vi "BuildPieceArrayFromPosition.vi"(8 "error in (no error)":errorcluster, 11 "object in":refnum<class "Board.lvclass">) -> (0 "error out":errorcluster, 3 "object out":refnum<class "Board.lvclass">)   [LabVIEW 2020, in "Board.lvclass"]
doc: "Returns a piece array from the board string"
uses:
  Board.lvclass
  Pieces/typedefs/pieceType.ctl
  Pieces/Piece.lvclass
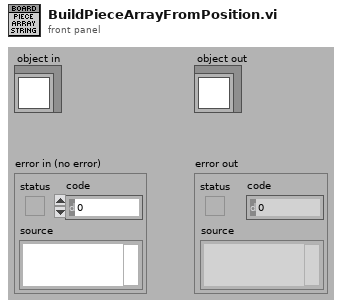
[diagram p1: front panel]
types:
  T1 = typedef "Piece.lvclass/pieceType.ctl" = enum16{"K", "Q", "R", "N", "B", "P", "none"}
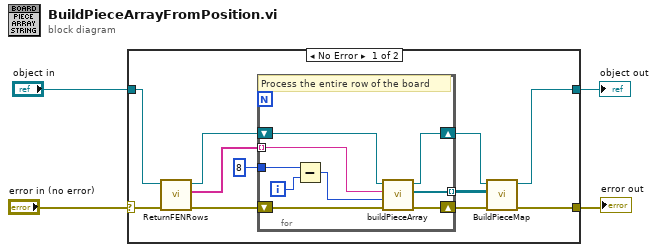
[diagram p0: block diagram]
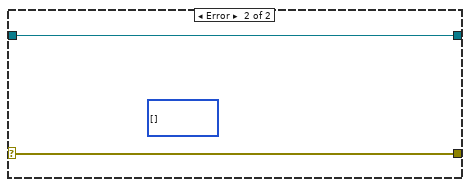
[diagram p2: hidden frame]
diagram:
  n1 = case shown="No Error" "error in (no error)" {
    selector: "error in (no error)" -> [w12 w26]
    tunnel: [w8 w26] -> w3
    tunnel: [w7 w25] -> w1
    tunnel: "object in" -> [w11 w25]
    frame No Error {
      n2 = call "ReturnFENRows.vi"("error in (no error)"=w12, "Board in"=w11) -> ("error out"=w13:errorcluster, "StandardPieceLocation"=w15:string[], "Board out"=w6:refnum<class "Board.lvclass">)  [unwired: 7 in]
      n3 = for {
        tunnel: w15 -> [w18] mode=indexing
        tunnel: [w20] -> w10 mode=indexing
        tunnel: 8 -> [w22]
        shift-right: [w23] -> w9
        shift-left: w13 -> [w24]
        shift-right: [w16] -> w5
        shift-left: w6 -> [w17]
        i -> [w21]
        # "Process the entire row of the board"
        n4 = Subtract(x=w22, y=w21) -> (x-y=w19:i32)
        n5 = call "buildPieceArray.vi"("error in (no error)"=w24, 9:"Row"=w19, 10:"Row"=w18, "object in"=w17) -> ("error out"=w23:errorcluster, "Piece array"=w20:refnum<class "Piece.lvclass">[], "object out"=w16:refnum<class "Board.lvclass">)  [unwired: 5 in]
      }
      n6 = call "BuildPieceMap.vi"("error in (no error)"=w9, "pieceArray"=w10, "object in"=w5) -> ("error out"=w8:errorcluster, "object out"=w7:refnum<class "Board.lvclass">)  [unwired: 7 in]
    }
    frame Error {
      (unwired) T1[][] [] items=["K", "Q", "R", "N", "B", "P", "none"] ("Pieces")
    }
  }
  "error out" <- w3
  "object out" <- w1
